vi "String to Double.vi"(11 "string":string) -> (3 "number":dbl)   [LabVIEW 2020, in "GOLPI library.lvlib"]
doc: "Converts string with real number into double format. In the case of parse error output is set to NaN."
uses:
  GOLPI library.lvlib
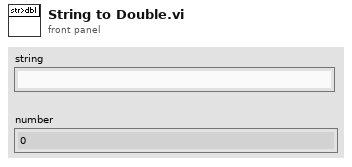
[diagram p1: front panel]
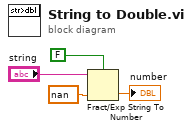
[diagram p0: block diagram]
diagram:
  n1 = Fract/Exp String To Number(use system decimal point (T)=FALSE, string="string", default (0 dbl)=nan ("default (0 DBL)")) -> (number=→"number":dbl)  [unwired: 1 in, 1 out]
